vi "SwerveModulePosition_CompareTo.vi"(9 "other SWERVE_DRIVE_MODULE_POSITION":T1={"Distance"=0.0, "Angle"={"VALUE"=0.0, "COS"=1.0, "SIN"=0.0}, "P"=FALSE} {"Angle"."SIN" format="%13.4f"; "Angle"."COS" format="%13.4f"; "Angle"."VALUE" format="%13.4f"}, 11 "in SWERVE_DRIVE_MODULE_POSITION":T1={"Distance"=0.0, "Angle"={"VALUE"=0.0, "COS"=1.0, "SIN"=0.0}, "P"=FALSE} {"Angle"."SIN" format="%13.4f"; "Angle"."COS" format="%13.4f"; "Angle"."VALUE" format="%13.4f"}) -> (3 "Compare":i32)   [LabVIEW 2019, in "Trajectory_Library.lvlib"]
doc: "Compares two swerve module positions. One swerve module is \"greater\" than the other if its position is higher than the other.\n\nParmeters:\n - this Module Position\n - other Module Position - The other swerve module.\n\nReturns:\n - compare - comparison result where\n 1 if this is greater, \n 0 if both are equal, \n -1 if other is greater."
uses:
  Trajectory_Library.lvlib
  TypeDef/ROTATION2D.ctl
  TypeDef/SWERVE_DRIVE_MODULE_POSITION.ctl
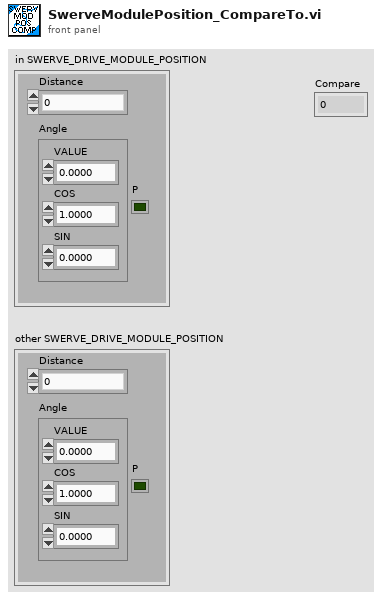
[diagram p1: front panel]
types:
  T1 = typedef "Trajectory_Library.lvlib/SWERVE_DRIVE_MODULE_POSITION.ctl" = cluster{"Distance":dbl, "Angle":T2, "P":bool}
  T2 = typedef "Trajectory_Library.lvlib/ROTATION2D.ctl" = cluster{"VALUE":dbl, "COS":dbl, "SIN":dbl}
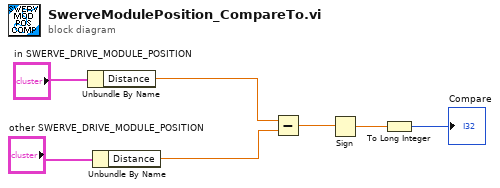
[diagram p0: block diagram]
diagram:
  n1 = Unbundle By Name("in SWERVE_DRIVE_MODULE_POSITION") -> ("Distance"=w5:dbl)
  n2 = Unbundle By Name("other SWERVE_DRIVE_MODULE_POSITION") -> ("Distance"=w4:dbl)
  n3 = Subtract(x=w5, y=w4) -> (x-y=w3:dbl)
  n4 = Sign(1:w3) -> (0:w2:dbl)
  n5 = To Long Integer(number=w2) -> (32bit integer=→"Compare":i32)
